vi "mod_D16 P005 filter design.vi"(1 "alias protect in final transition":bool, 2 "stop band attenuation":T1(ring)=enum."72 dB") -> (0 "h":dbl[](array[numeric]) format="%.2f")   [LabVIEW 2020, in "niAMT.lvlib"]
uses:
  <vilib>/addons/Modulation/niAMT.lvlib
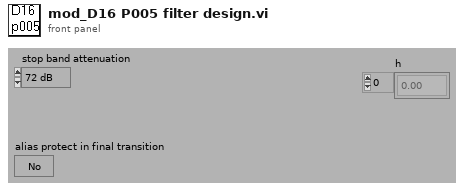
[diagram p1: front panel]
types:
  T1 = enum16{"48 dB", "60 dB", "72 dB", "84 dB", "96 dB", "120 dB"}
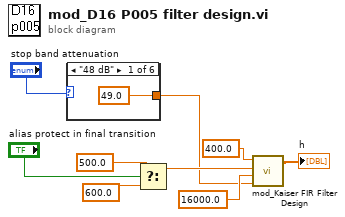
[diagram p0: block diagram]
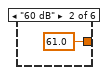
[diagram p2: hidden frame]
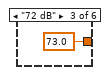
[diagram p3: hidden frame]
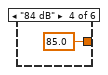
[diagram p4: hidden frame]
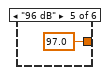
[diagram p5: hidden frame]
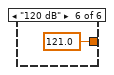
[diagram p6: hidden frame]
diagram:
  n1 = case shown="\"48 dB\"" "stop band attenuation" {
    tunnel: [49.0 61.0 73.0 85.0 97.0 121.0] -> w2
    frame "48 dB" {
    }
    frame "60 dB" {
    }
    frame "72 dB" {
    }
    frame "84 dB" {
    }
    frame "96 dB" {
    }
    frame "120 dB" {
    }
  }
  n2 = Select(t=500.0 ("high cutoff freq: fh"), s="alias protect in final transition", f=600.0 ("high cutoff freq: fh")) -> (s? t:f=w4:dbl)
  n3 = call <vilib>:"mod_Kaiser FIR Filter Design.vi"("Stop Attenuation"=w2, "sampling freq: fs"=16000.0, "high cutoff freq: fh"=w4, "low cutoff freq: fl"=400.0) -> ("h"=→"h":dbl[])  [unwired: 1 out]
